vi "Create Collection.vi"(10 "Cache":refnum<class "ConfigManager.Cache.lvclass">, 11 "List":refnum<class "ConfigManager.lvclass">[](array[class])) -> (3 "ConfigManagerCollection out":refnum<class "ConfigManagerCollection.lvclass">)   [LabVIEW 2013, in "CfgManager.lvlib" / "ConfigManagerCollection.lvclass"]
uses:
  ConfigManagerCollection.lvclass
  Manager/ConfigManager.lvclass
  Cache/ConfigManager.Cache.lvclass
  ConfigManagerCollection.lvclass/ConfigManagerCollection.ctl
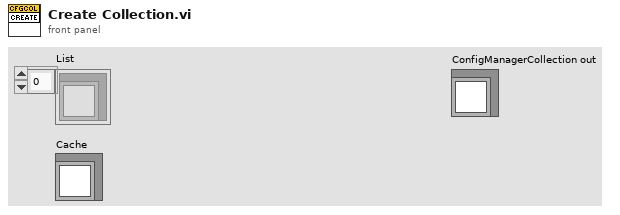
[diagram p1: front panel]
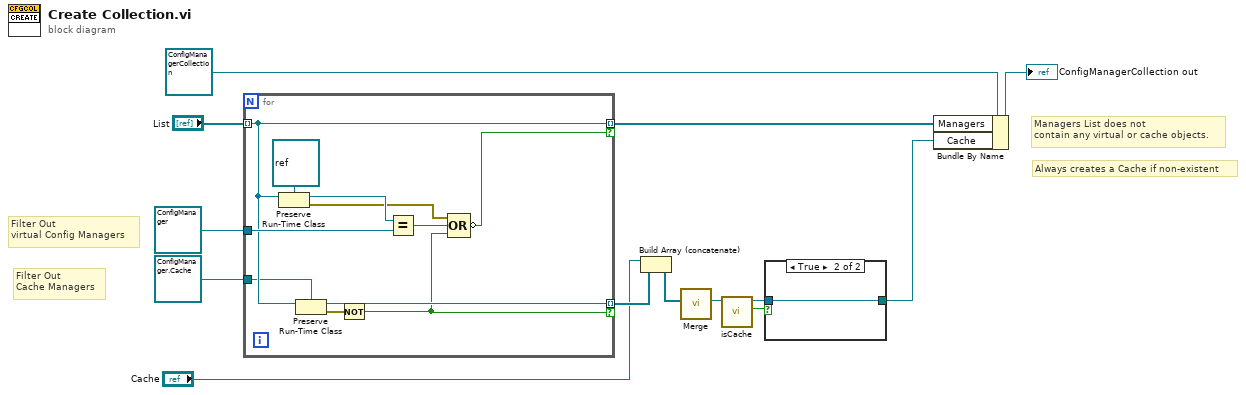
[diagram p0: block diagram]
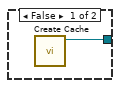
[diagram p2: hidden frame]
diagram:
  # "Always creates a Cache if non-existent"
  # "Managers List does not\ncontain any virtual or cache objects."
  # "Filter Out\nCache Managers"
  # "Filter Out\nvirtual Config Managers"
  n1 = for {
    tunnel: "List" -> [w18] mode=indexing
    tunnel: refnum<class "ConfigManager.lvclass"> refnum ("ConfigManager.lvclass") -> [w24]
    tunnel: [w18] -> w9 mode=indexing if=w20
    tunnel: [w15] -> w8 mode=indexing if=w14
    tunnel: refnum<class "ConfigManager.Cache.lvclass"> refnum ("Config.lvlib:ConfigManager.Cache.lvclass") -> [w16]
    n2 = Preserve Run-Time Class(object in=w18, 2:refnum<class> refnum ("LabVIEW Object")) -> (object out=w22:refnum<class>, error out=w19:errorcluster)  [unwired: 1 in]
    n3 = Preserve Run-Time Class(object in=w18, 2:w16) -> (object out=w15:refnum<class "ConfigManager.Cache.lvclass">, error out=w17:errorcluster)  [unwired: 1 in]
    n4 = Not(x=w17) -> (.not. x?=w14:bool)
    n5 = Equal?(x=w22, y=w24) -> (x = y?=w21:bool)
    n6 = Compound Arithmetic op=OR(w19, w21, w14) -> (invert w20:bool)
  }
  n7 = Build Array (concatenate)("Cache", w8) -> (w3:refnum<class "ConfigManager.Cache.lvclass">[])
  n8 = call "Merge.vi"("Cache Managers"=w3) -> ("Merged Cache"=w6:refnum<class "ConfigManager.Cache.lvclass">)  [unwired: 10 in]
  n9 = call "isCache.vi"("ConfigManager.Cache in"=w6) -> ("isCache?"=w5:bool, "ConfigManager.Cache out"=w4:refnum<class "ConfigManager.Cache.lvclass">)  [unwired: 9 in]
  n10 = case shown="True" w5 {
    tunnel: [w25 w26] -> w7
    tunnel: w4 -> [_ w26]
    frame False {
      n11 = call "Create Cache.vi"() -> ("ConfigManager.Cache"=w25:refnum<class "ConfigManager.Cache.lvclass">)  [unwired: 11 in]
    }
    frame True {
    }
  }
  n12 = Bundle By Name(cluster=refnum<class "ConfigManagerCollection.lvclass"> refnum ("ConfigManagerCollection.lvclass"), "Managers"=w9, "Cache"=w7) -> (→"ConfigManagerCollection out":refnum<class "ConfigManagerCollection.lvclass">)
